vi "RT_VS50_Dynamics_DLR.vi"() -> ()   [LabVIEW 2017]
uses:
  <vilib>/Platform/TimedLoop/XDataNode/timing_clust.ctl
  <vilib>/Platform/TimedLoop/XDataNode/nitl_modes.ctl
  <vilib>/Platform/TimedLoop/XDataNode/wakeup.ctl
  <vilib>/Analysis/coordinate.llb/Euler Rotation Order.ctl
  <vilib>/Analysis/baseanly.llb/Real A x B.vi
  <vilib>/Utility/file.llb/Read Delimited Spreadsheet (DBL).vi
  <vilib>/Analysis/Matrix/Numeric/Conversions/Array To Matrix - RA.vi
  <vilib>/Analysis/Matrix/Numeric/Conversions/Array To Matrix - RA2.vi
  <vilib>/Analysis/Matrix/Numeric/Conversions/Matrix To Array - RM.vi
  <vilib>/platform/TimedLoop/XDataNode/XDataNode.xnode
  <vilib>/Platform/TimedLoop/XDataNode/XDNodeRunTimeDep.lvlib
  <vilib>/Analysis/Matrix/NI_Matrix.lvlib
  <vilib>/Analysis/NI_AALBase.lvlib
  <vilib>/Analysis/NI_AALPro.lvlib
panel:
  out "M_beta":dbl
  out "M_alpha":dbl
  out "TVA_cmd [rad]":dbl[](array[numeric])
  in  "TVA_y [º]":dbl=-0.01 format="%#_13g"
  in  "TVA_p [º]":dbl=-0.01 format="%#_13g"
  out "Sref [m^2]":dbl
  out "MAd [Nm]":dbl[](array[numeric])
  out "MA_f [Nm]":dbl[](array[numeric])
  out "TVA_b":dbl[](array[numeric])
  out "P(i) [m/s]":dbl[](array[numeric])
  out "MFE_b":dbl[](array[numeric])
  out "Euler Angles [º]":cluster{"phi":dbl, "theta":dbl, "psi":dbl}
  out "Euler Angles [rad]":cluster{"phi":dbl, "theta":dbl, "psi":dbl}
  out "Waveform Chart":T1(graph)
  out "alt(i)":dbl
  out "alt(i+1)":dbl
  out "lon(i)":dbl
  out "latd(i)":dbl
  out "lon(i+1)":dbl
  out "latd(i+1)":dbl
  out "R_lh [m]":dbl
  out "R_l [m]":dbl
  out "L_C [rad]":dbl
  out "D_l [rad]":dbl
  out "W_b(i) [º/s]":dbl[](array[numeric])
  out "q(i)":dbl[](array[numeric])
  out "W(i)":dbl[](array[numeric])
  out "V(i+1)":dbl[](array[numeric])
  out "V(i) [m/s]":dbl[](array[numeric])
  out "W(i+1)":dbl[](array[numeric])
  out "q(i+1)":dbl[](array[numeric])
  out "z(i)":dbl[](array[numeric])
  out "y(i)":dbl[](array[numeric])
  out "x(i)":dbl[](array[numeric])
  out "z(i+1)":dbl[](array[numeric])
  out "y(i+1)":dbl[](array[numeric])
  out "x(i+1)":dbl[](array[numeric])
  out "t [s]":dbl
  out "dt[s]":dbl
  in  "Tempo total de simulação":i32=85
  out "ang_acc [rad/s^2]":dbl[](array[numeric])
  out "acc [m/s^2]":dbl[](array[numeric])
  out "MFA [Nm]":dbl[](array[numeric])
  out "MFE [Nm]":dbl[](array[numeric])
  out "Mco [Nm]":dbl[](array[numeric])
  out "Fco [N]":dbl[](array[numeric])
  out "FA [N]":dbl[](array[numeric])
  out "FG_b [N]":dbl[](array[numeric])
  out "FG [N]":dbl[](array[numeric])
  out "FE [N]":dbl[](array[numeric])
  out "FE_b [N]":dbl[](array[numeric])
  out "AoA_yaw [rad]":dbl
  out "AoA_pitch [rad]":dbl
  out "Iteration Duration":i64(graph)
  out "Patm [Pa]":dbl
  out "Pdin [Pa]":dbl
  out "Nzl_S [m^2]":dbl
  out "Data":dbl[][](array[numeric])
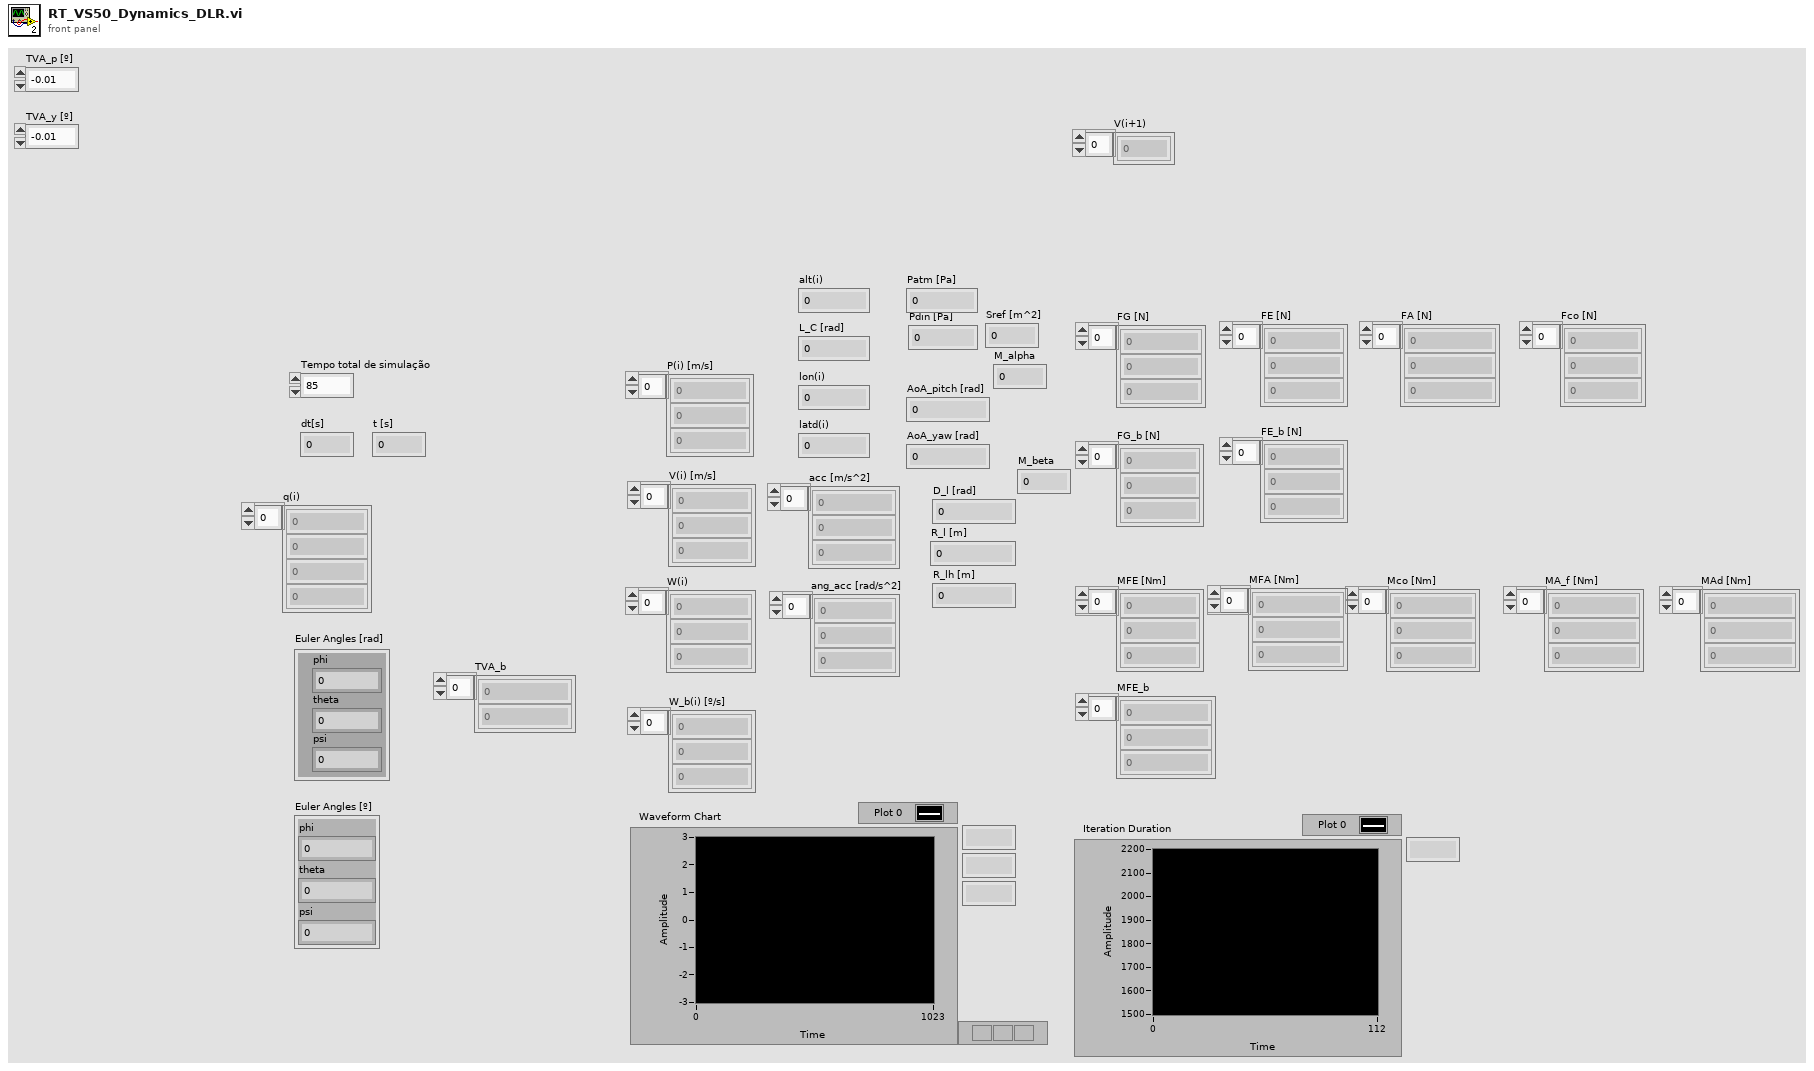
[diagram p1: front panel]
types:
  T1 = cluster{"Real Matrix Element":dbl, "Real Matrix Element":dbl, "Real Matrix Element":dbl}
  T2 = typedef "XDNodeRunTimeDep.lvlib/timing_clust.ctl" = cluster{"Expected End [f-1]":u64, "Actual End [f-1]":u64, "Finished Late? [f-1]":bool, "Expected End [i-1]":u64, "Actual End [i-1]":u64, "Finished Late? [i-1]":bool, "Expected Start [i]":u64, "Actual Start [i]":u64, "Expected Start [f]":u64, "Actual Start [f]":u64, "Source Name":string, "Structure Name":string, "Period":i64, "Deadline":i64, "Offset":i64, "Start":i64, "Priority":i32, "Timeout":i32, "Mode":T3, "Wakeup Reason":T4, "Error":errorcluster, "Source Type":string, "Secondary Source Type":string, "Global End Time":u64, "Global Start Time":u64, "Frame Duration":u64, "Iteration Duration":u64, "Assigned CPU":i32, "I/O Scan Engine Mode":u32}
  T3 = typedef "XDNodeRunTimeDep.lvlib/nitl_modes.ctl" = enum32{"No Change", "Process missed periods, maintain original phase", "Discard missed periods, maintain original phase", "Process missed periods, ignore original phase", "Discard missed periods, ignore original phase"}
  T4 = typedef "XDNodeRunTimeDep.lvlib/wakeup.ctl" = enum32{"Normal", "Aborted", "Asynchronous wakeup", "Timing source error", "Timed loop error", "Timeout"}
  T5 = typedef "NI_AALPro.lvlib/Euler Rotation Order.ctl" = u16
  T6 = typedef "NI_Matrix.lvlib/RealMatrix.ctl" = dbl[][]
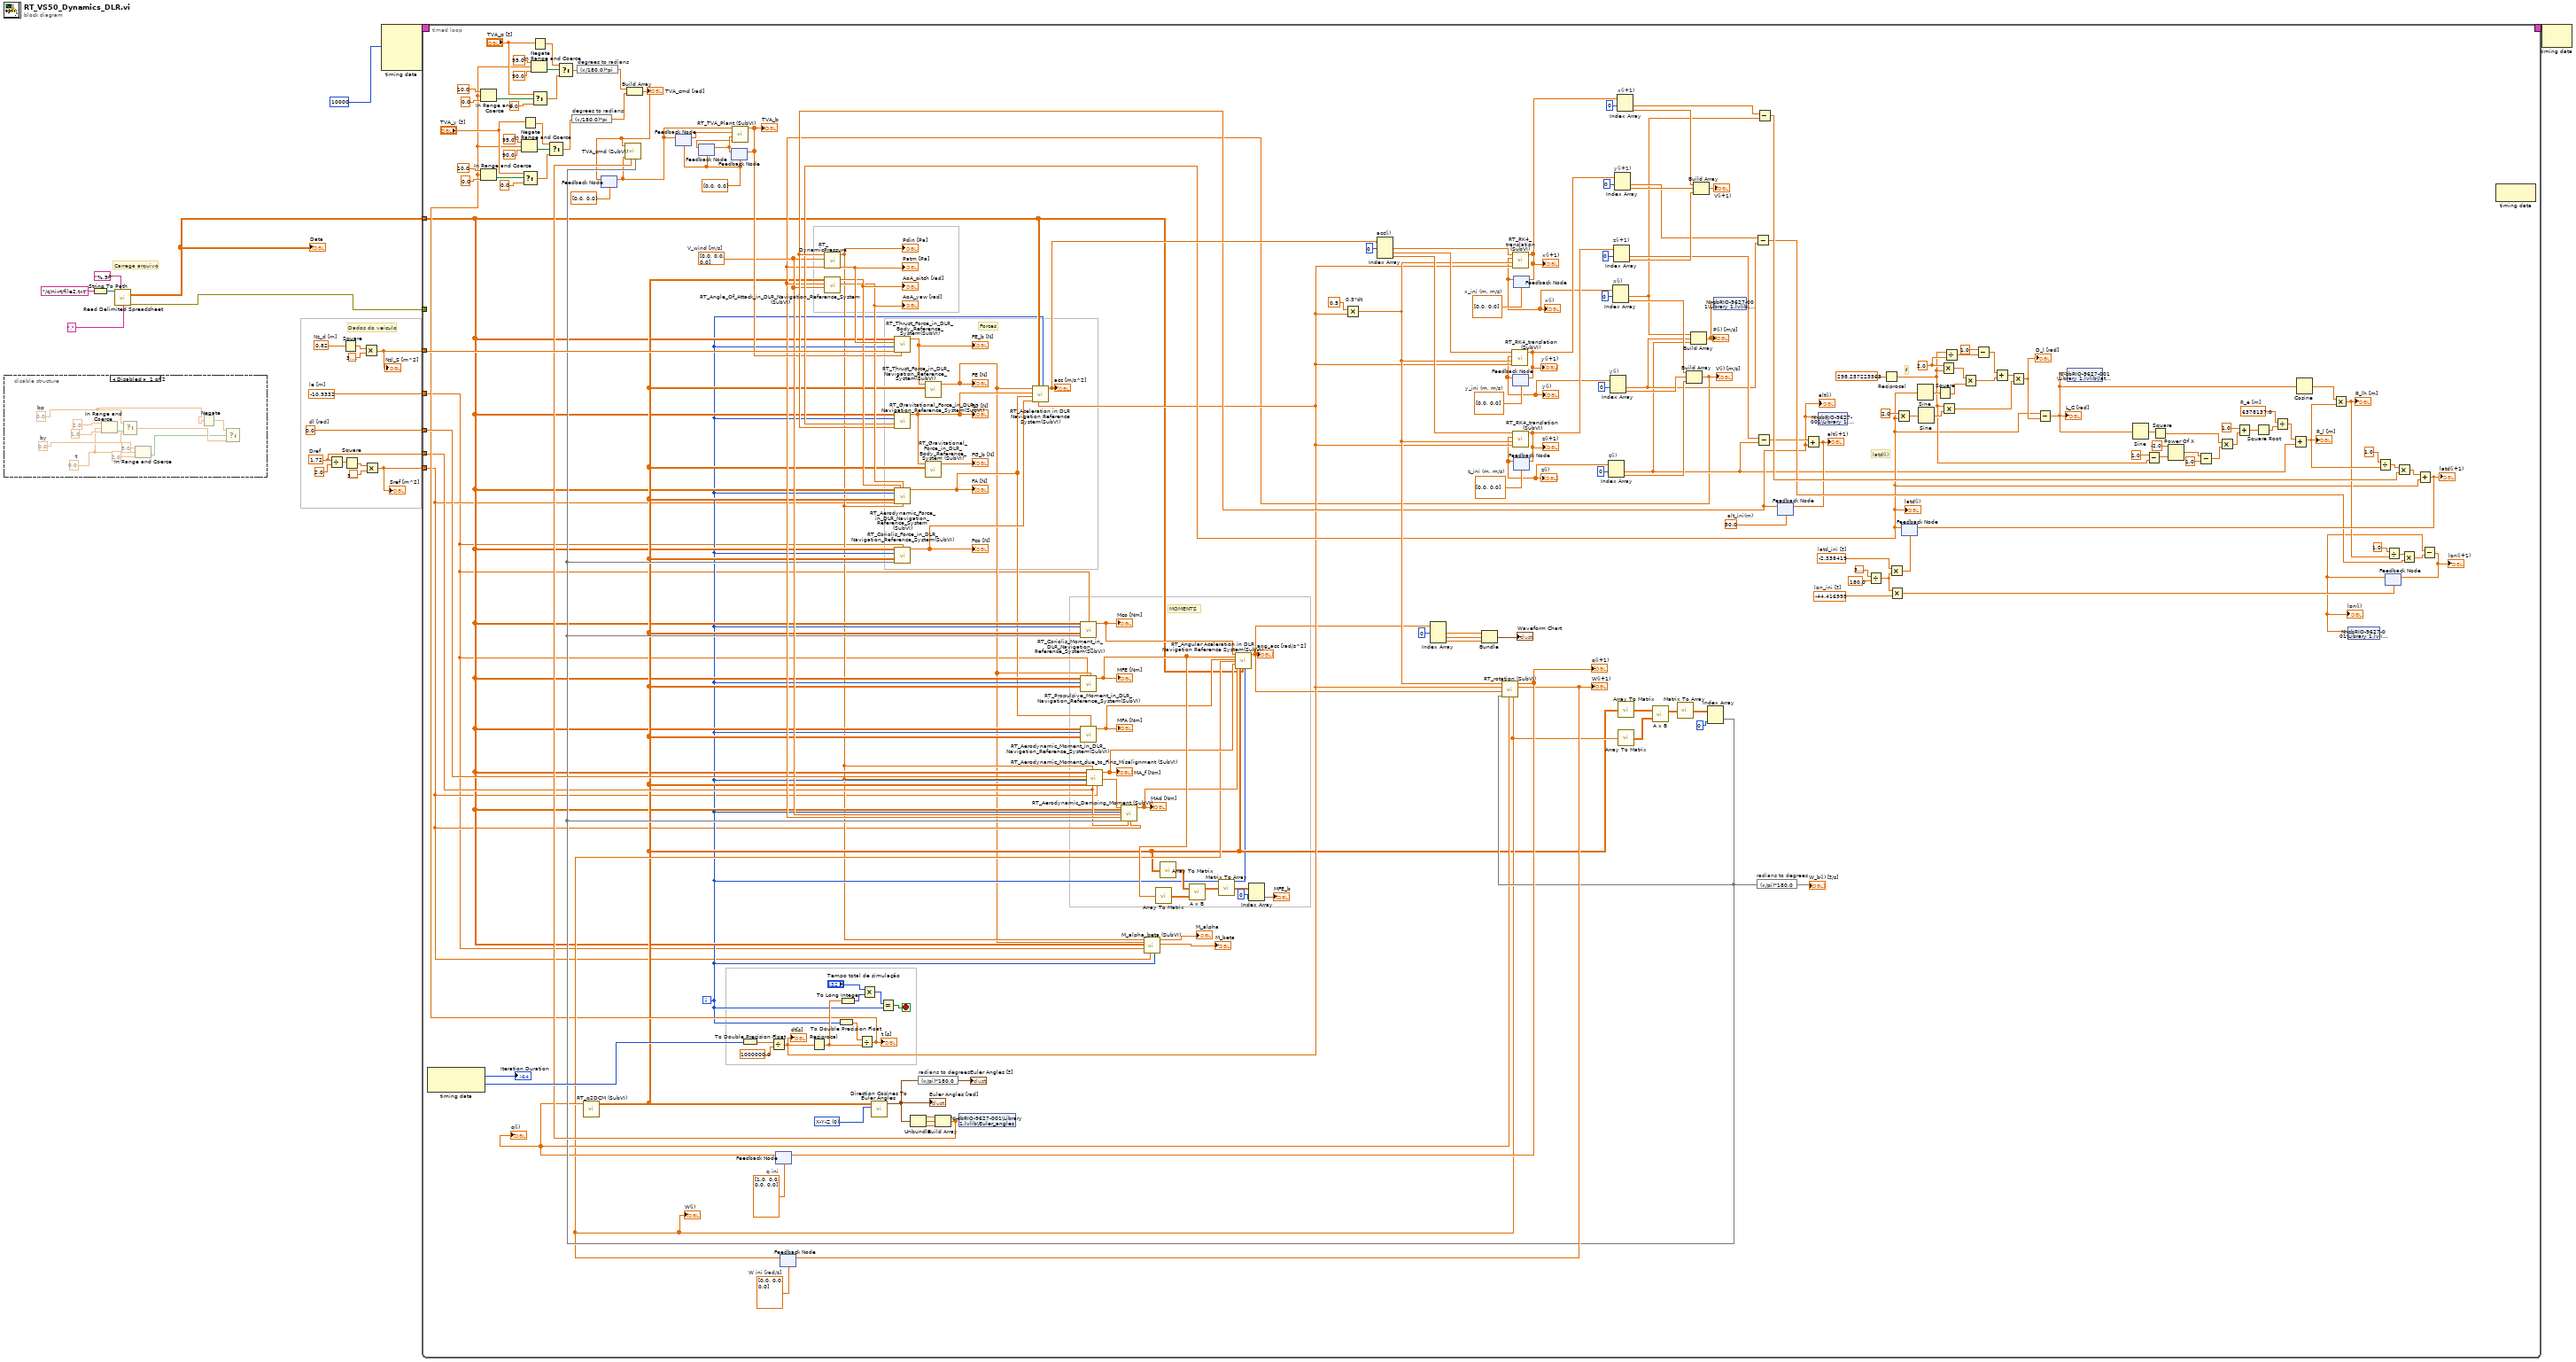
[diagram p0: block diagram]
diagram:
  w1 = 1.72  # Dref
  w7 = 0.0  # dl [rad]
  w14 = 0.82  # Nz_d [m]
  w15 = -10.9332  # le [m]
  # "Carrega arquivo"
  # "Dados do veículo"
  n1 = disable-structure shown="Disabled" {
    frame Disabled {
      w23 = 0.0  # t
      w24 = 0.0  # by
      w22 = 0.0  # bp
      n2 = In Range and Coerce(upper limit=2.0, x=w23, lower limit=1.0 ("y")) -> (In Range?=w31:bool)  [unwired: 1 out]
      n3 = Select(t=w22, s=w31, f=w24) -> (s? t:f=w27:dbl)
      n4 = In Range and Coerce(upper limit=3.0, x=w23, lower limit=2.0) -> (In Range?=w25:bool)  [unwired: 1 out]
      n5 = Negate(x=w22) -> (-x=w28:dbl)
      n6 = Select(t=w28, s=w25, f=w27) -> ()  [unwired: 1 out]
    }
    frame Enabled {
    }
  }
  n7 = String To Path(string="/c/ni-rt/file2.txt") -> (path=w18:path)
  n8 = call-poly <vilib>:"Read Delimited Spreadsheet.vi"("file path (dialog if empty)"=w18, "format (%.3f)"="%.9f", "delimiter (\\t)"="," ("delimiter (\\t)")) -> ("all rows"=w8:dbl[][], "error out"=w11:errorcluster)  [unwired: 7 in, 4 out]
  "Data" <- w8
  n9 = Divide(x=w1, y=2.0) -> (x/y=w3:dbl)
  n10 = Square(x=w14) -> (x^2=w17:dbl)
  n11 = Square(x=w3) -> (x^2=w4:dbl)
  n12 = Multiply(x=w17, y=3.141592653589793) -> (x*y=w13:dbl)
  "Nzl_S [m^2]" <- w13
  n13 = Multiply(x=w4, y=3.141592653589793) -> (x*y=w2:dbl)
  "Sref [m^2]" <- w2
  n14 = node-c288(i64 10000 ("Period")) -> (w21:T2)  [unwired: 3 in]
  n15 = timed-loop {
    timing: w21 -> [_]
    timing-out: [_] -> w20
    tunnel: w8 -> [w41]
    tunnel: w15 -> [w35]
    tunnel: w13 -> [w225]
    tunnel: w11 -> [_]
    tunnel: w7 -> [w83]
    tunnel: w2 -> [w38]
    tunnel: w1 -> [w43]
    i -> [w40]
    stop <- w227 stop-if-true
    w115 = T5 0 items=["X-Y-Z", "X-Z-Y", "Y-X-Z", "Y-Z-X", "Z-X-Y", "Z-Y-X", "X-Y-X", "X-Z-X", "Y-X-Y", "Y-Z-Y", "Z-X-Z", "Z-Y-Z"] ("rotation order")
    w89 = dbl[] [0.0, 0.0] ("TVA_b")
    w130 = 50.0  # alt_ini(m)
    w170 = 2.0 ("x")
    w150 = 6378137.0  # R_e [m]
    w82 = dbl[] [0.0, 0.0, 0.0]  # V_wind [m/s]
    w181 = -44.416995  # lon_ini [º]
    w183 = -2.338419  # latd_ini [º]
    w206 = dbl[] [0.0, 0.0]  # z_ini (m, m/s)
    w126 = dbl[] [0.0, 0.0, 0.0]  # W ini [rad/s]
    w207 = dbl[] [0.0, 0.0]  # y_ini (m, m/s)
    w210 = dbl[] [0.0, 0.0]  # x_ini (m, m/s)
    w127 = dbl[] [1.0, 0.0, 0.0, 0.0]  # q ini
    # "MOMENTS"
    # "Forces"
    # "f"
    # "latd(i)"
    n16 = node-c288() -> (→"Iteration Duration":i64, w216:i64)  [unwired: 1 in]
    n17 = Negate(x="TVA_y [º]") -> (-x=w49:dbl)
    n18 = Negate(x="TVA_p [º]") -> (-x=w70:dbl)
    n19 = feedback #1(dbl[] [0.0, 0.0] ("TVA_cmd")) -> (w44:dbl[])
    n20 = feedback #2(w89) -> (w88:dbl[])
    n21 = feedback-in #2(w44) -> ()
    n22 = feedback #3(w89) -> (w85:dbl[])
    n23 = feedback #4(w89) -> (w86:dbl[])
    n24 = feedback-in #3(w86) -> ()
    n25 = call "RT_TVA_Plant (SubVI).vi"("TVA_b(i-2)"=w85, "TVA_b(i-1)"=w86, "TVA_cmd (i-2) [rad]"=w88, "TVA_cmd (i-1) [rad]"=w44) -> ("TVA_b"=w87:dbl[])  [unwired: 7 in]
    "TVA_b" <- w87
    n26 = feedback-in #4(w87) -> ()
    n27 = To Double Precision Float(number=w216) -> (double precision float=w215:dbl)
    n28 = Divide(x=w215, y=1000000.0) -> (x/y=w117:dbl)
    "dt[s]" <- w117
    n29 = feedback #5(w127) -> (w79:dbl[])
    "q(i)" <- w79
    n30 = call "RT_q2DCM (SubVI).vi"("Quaternion"=w79) -> ("DCM"=w42:dbl[][])  [unwired: 10 in]
    n31 = feedback #6(w126) -> (w72:dbl[])
    "W(i)" <- w72
    n32 = Reciprocal(x=w117) -> (1/x=w187:dbl)
    n33 = To Double Precision Float(number=w40) -> (double precision float=w186:dbl)
    n34 = To Long Integer(number=w187) -> (32bit integer=w213:i32)
    n35 = Divide(x=w186, y=w187) -> (x/y=w46:dbl)
    "t [s]" <- w46
    n36 = In Range and Coerce(upper limit=10.0, x=w46, lower limit=0.0) -> (In Range?=w64:bool)  [unwired: 1 out]
    n37 = In Range and Coerce(upper limit=10.0, x=w46, lower limit=0.0) -> (In Range?=w52:bool)  [unwired: 1 out]
    n38 = In Range and Coerce(upper limit=95.0, x=w46, lower limit=90.0) -> (In Range?=w51:bool)  [unwired: 1 out]
    n39 = Select(t="TVA_y [º]", s=w52, f=0.0 ("t")) -> (s? t:f=w50:dbl)
    n40 = In Range and Coerce(upper limit=95.0, x=w46, lower limit=90.0) -> (In Range?=w65:bool)  [unwired: 1 out]
    n41 = Select(t="TVA_p [º]", s=w64, f=0.0 ("t")) -> (s? t:f=w67:dbl)
    n42 = Select(t=w49, s=w51, f=w50) -> (s? t:f=w47:dbl)
    n43 = Select(t=w70, s=w65, f=w67) -> (s? t:f=w66:dbl)
    n44 = expression code="(x/180.0)*pi" "degrees to radians"(w47) -> (w69:dbl)
    n45 = expression code="(x/180.0)*pi" "degrees to radians"(w66) -> (w68:dbl)
    n46 = Build Array(w68, w69) -> (w45:dbl[])
    "TVA_cmd [rad]" <- w45
    n47 = feedback-in #1(w45) -> ()
    n48 = Multiply(x="Tempo total de simulação", y=w213) -> (x*y=w228:i32)
    n49 = call <vilib>:"Direction Cosines To Euler Angles.vi"("rotation order"=w115, "Direction Cosines"=w42) -> ("Euler Angles"=w111:cluster{"phi":dbl, "theta":dbl, "psi":dbl})  [unwired: 8 in, 1 out]
    "Euler Angles [rad]" <- w111
    n50 = Equal?(x=w228, y=w40) -> (x = y?=w227:bool)
    n51 = Unbundle(w111) -> ("phi"=w114:dbl, "theta"=w112:dbl, "psi"=w113:dbl)
    n52 = expression code="(x/pi)*180.0" "radians to degrees"(w111) -> (→"Euler Angles [º]":cluster{"phi":dbl, "theta":dbl, "psi":dbl})
    n53 = Build Array(w114, w112, w113) -> (w90:dbl[])
    n54 = shared-variable "NI-sbRIO-9627-001\\Library 1.lvlib\\Euler_angles"(w90) -> ()  [unwired: 1 in, 1 out]
    n55 = call-poly <vilib>:"Array To Matrix.vi"("Real 2D Array"=w42) -> ("Real Matrix"=w98:T6)
    n56 = Multiply "0.5*dt"(x=0.5, y=w117) -> (x*y=w204:dbl)
    n57 = feedback #7(w207) -> (w96:dbl[])
    "y(i)" <- w96
    n58 = feedback #8(w210) -> (w97:dbl[])
    "x(i)" <- w97
    n59 = feedback #9(w206) -> (w95:dbl[])
    "z(i)" <- w95
    n60 = Index Array "z(i)"(array=w95, index #1=0 ("index")) -> (element #1=w92:dbl, element #2=w116:dbl)  [unwired: 1 in]
    n61 = Index Array "y(i)"(array=w96, index #1=0 ("index")) -> (element #1=w93:dbl, element #2=w198:dbl)  [unwired: 1 in]
    n62 = Index Array "x(i)"(array=w97, index #1=0 ("index")) -> (element #1=w94:dbl, element #2=w199:dbl)  [unwired: 1 in]
    n63 = call-poly <vilib>:"Array To Matrix.vi"("Real 2D Array"=w42) -> ("Real Matrix"=w125:T6)
    n64 = call-poly <vilib>:"Array To Matrix.vi"("Real 1D Array"=w72) -> ("Real Matrix (Column Vector)"=w124:T6)
    n65 = call-poly <vilib>:"A x B.vi"("B"=w124, "A"=w125) -> ("A x B"=w122:T6)  [unwired: 1 out]
    n66 = call-poly <vilib>:"Matrix To Array.vi"("Real Matrix"=w122) -> ("Real 2D Array"=w123:dbl[][])
    n67 = Build Array(w199, w198, w116) -> (w81:dbl[])
    "V(i) [m/s]" <- w81
    n68 = call "RT_Angle_Of_Attack_in_DLR_Navigation_Reference_System (SubVI).vi"("V_wind (m/s)"=w82, "V (m/s)"=w81, "DCM"=w42) -> ("AoA_yaw (rad)"=w221:dbl, "AoA_pitch (rad)"=w222:dbl)  [unwired: 7 in]
    "AoA_pitch [rad]" <- w222
    "AoA_yaw [rad]" <- w221
    n69 = Build Array(w94, w93, w92) -> (w71:dbl[])
    "P(i) [m/s]" <- w71
    n70 = Index Array(array=w123, index (col)=0 ("index (row)")) -> (element=w80:dbl[])  [unwired: 1 in]
    n71 = call "TVA_cmd (SubVI).vi"("W_b [rad/s]"=w80, "Angles [rad]"=w90, "TVA_old [rad]"=w44, "TVA_cmd [rad]"=w45) -> ()  [unwired: 6 in, 2 out]
    n72 = call "RT_Coriolis_Force_in_DLR_Navigation_Reference_System(SubVI).vi"("Data"=w41, "le (m) in"=w35, "i"=w40, "DCM"=w42, "W_b (rad/s)"=w80) -> ("Fco (N)"=w220:dbl[])  [unwired: 10 in]
    "Fco [N]" <- w220
    n73 = call "RT_Coriolis_Moment_in_DLR_Navigation_Reference_System(SubVI).vi"("Data"=w41, "le (m) in"=w35, "i"=w40, "DCM"=w42, "W_b (rad/s) in"=w80) -> ("Mco (Nm)"=w77:dbl[])  [unwired: 10 in]
    "Mco [Nm]" <- w77
    n74 = shared-variable "NI-sbRIO-9627-001\\Library 1.lvlib\\Pos"(w71) -> ()  [unwired: 1 in, 1 out]
    n75 = expression code="(x/pi)*180.0" "radians to degrees"(w80) -> (→"W_b(i) [º/s]":dbl[])
    n76 = feedback #10(w130) -> (w120:dbl)
    "alt(i)" <- w120
    n77 = call "RT_DynamicPressure.vi"("V (m/s)"=w81, "V_wind (m/s)"=w82, "h (m)"=w120) -> ("Patm (Pa)"=w223:dbl, "Pdin"=w39:dbl)  [unwired: 7 in]
    "Pdin [Pa]" <- w39
    "Patm [Pa]" <- w223
    n78 = call "RT_Thrust_Force_in_DLR_Body_Reference_System(SubVI).vi"("TVA_b(i)"=w87, "Nzl_S"=w225, "i"=w40, "Patm (Pa)"=w223, "Data"=w41) -> ("FE_b"=w104:dbl[])  [unwired: 6 in]
    "FE_b [N]" <- w104
    n79 = call "RT_Aerodynamic_Force_in_DLR_Navigation_Reference_System (SubVI).vi"("Data"=w41, "AoA_pitch (rad)"=w222, "AoA_yaw (rad)"=w221, "i"=w40, "DCM"=w42, "Sref [m^2]"=w38, "Pdin"=w39) -> ("FA"=w37:dbl[])  [unwired: 8 in]
    "FA [N]" <- w37
    n80 = call "RT_Thrust_Force_in_DLR_Navigation_Reference_System(SubVI).vi"("DCM"=w42, "FE_b"=w104) -> ("FE"=w36:dbl[])  [unwired: 8 in]
    "FE [N]" <- w36
    n81 = call "RT_Propulsive_Moment_in_DLR_Navigation_Reference_System(SubVI).vi"("FE"=w36, "le (m) in"=w35, "DCM"=w42, "i"=w40, "Data"=w41) -> ("MFE (Nm)"=w76:dbl[])  [unwired: 6 in]
    "MFE [Nm]" <- w76
    n82 = call "RT_Aerodynamic_Moment_in_DLR_Navigation_Reference_System(SubVI).vi"("FA"=w37, "DCM"=w42, "i"=w40, "Data"=w41) -> ("MFA (Nm)"=w75:dbl[])  [unwired: 7 in]
    "MFA [Nm]" <- w75
    n83 = call "RT_Aerodynamic_Moment_due_to_Fins_Misalignment (SubVI).vi"("Sref [m^2]"=w38, "Dref"=w43, "Pdin [Pa]"=w39, "DCM"=w42, "i"=w40, "dl [rad] in"=w83, "Data"=w41) -> ("MA_f"=w74:dbl[])  [unwired: 4 in]
    "MA_f [Nm]" <- w74
    n84 = call "RT_Aerodynamic_Damping_Moment (SubVI).vi"("Pdin [Pa]"=w39, "Data"=w41, "i"=w40, "V_wind [m/s]"=w82, "V(i) [m/s]"=w81, "W_b(i) [º/s]"=w80, "Dref"=w43, "Sref [m^2]"=w38) -> ("MAd"=w73:dbl[])  [unwired: 11 in]
    "MAd [Nm]" <- w73
    n85 = call "M_alpha_beta (SubVI).vi"("i"=w40, "Sref"=w38, "FE [N]"=w36, "le [m]"=w35, "Data"=w41, "Pdin [Pa]"=w39) -> ("M_beta"=→"M_beta":dbl, "M_alpha"=→"M_alpha":dbl)  [unwired: 4 in]
    n86 = call-poly <vilib>:"Array To Matrix.vi"("Real 1D Array"=w76) -> ("Real Matrix (Column Vector)"=w103:T6)
    n87 = call-poly <vilib>:"A x B.vi"("B"=w103, "A"=w98) -> ("A x B"=w101:T6)  [unwired: 1 out]
    n88 = call-poly <vilib>:"Matrix To Array.vi"("Real Matrix"=w101) -> ("Real 2D Array"=w102:dbl[][])
    n89 = call "RT_Angular Aceleration in DLR Navigation Reference System(SubVI).vi"("Mco (Nm)"=w77, "MFE (Nm)"=w76, "MFA (Nm)"=w75, "W (rad/s)"=w72, "MA_f [Nm]"=w74, "MAd [Nm]"=w73, "DCM"=w42, "Data"=w41, "i"=w40) -> ("ang_acc"=w78:dbl[])  [unwired: 10 in]
    "ang_acc [rad/s^2]" <- w78
    n90 = Index Array(array=w102, index (col)=0 ("index (row)")) -> (element=→"MFE_b":dbl[])  [unwired: 1 in]
    n91 = Index Array(array=w78, index #1=0 ("index")) -> (element #1=w108:dbl, element #2=w106:dbl, element #3=w107:dbl)  [unwired: 2 in]
    n92 = Bundle("Real Matrix Element"=w108, "Real Matrix Element"=w106, "Real Matrix Element"=w107) -> (→"Waveform Chart":T1)  [unwired: 1 in]
    n93 = call "RT_rotation (SubVI).vi"("W(i) (rad/s) in"=w72, "q(i) in"=w79, "W_b(i)"=w80, "ang_acc"=w78, "dt"=w117, "dt*0.5"=w204) -> ("W(i+1)"=w84:dbl[], "q(i+1)"=w203:dbl[])  [unwired: 4 in]
    "q(i+1)" <- w203
    "W(i+1)" <- w84
    n94 = feedback-in #5(w203) -> ()
    n95 = feedback-in #6(w84) -> ()
    n96 = shared-variable "NI-sbRIO-9627-001\\Library 1.lvlib\\alt"(w120) -> ()  [unwired: 1 in, 1 out]
    n97 = Divide(x=3.141592653589793, y=180.0) -> (x/y=w182:dbl)
    n98 = Reciprocal(x=298.257223563) -> (1/x=w161:dbl)
    n99 = Multiply(x=w183, y=w182) -> (x*y=w179:dbl)
    n100 = Multiply(x=w182, y=w181) -> (x*y=w178:dbl)
    n101 = feedback #11(w179) -> (w119:dbl)
    "latd(i)" <- w119
    n102 = call "RT_Gravitational_Force_in_DLR_Navigation_Reference_System(SubVI).vi"("Data"=w41, "i"=w40, "latd (rad)"=w119, "alt (m)"=w120) -> ("FG_d"=w218:dbl[])  [unwired: 10 in, 1 out]
    "FG [N]" <- w218
    n103 = call "RT_Gravitational_Force_in_DLR_Body_Reference_System (SubVI).vi"("DCM"=w42, "FG_d"=w218) -> ("FG_b"=→"FG_b [N]":dbl[])  [unwired: 9 in]
    n104 = call "RT_Aceleration in DLR Navigation Reference System(SubVI).vi"("i"=w40, "dt(s)"=w117, "Data"=w41, "Fco (N)"=w220, "FA"=w37, "FG"=w218, "FE"=w36) -> ("acc"=w212:dbl[])  [unwired: 4 in]
    "acc [m/s^2]" <- w212
    n105 = Index Array "acc(i)"(array=w212, index #1=0 ("index")) -> (element #1=w209:dbl, element #2=w208:dbl, element #3=w205:dbl)  [unwired: 2 in]
    n106 = call "RT_RK4_translation (SubVI).vi"("dt"=w117, "dt*0.5"=w204, "x(i)"=w96, "accx"=w208) -> ("x(i+1)"=w193:dbl[])  [unwired: 7 in]
    "y(i+1)" <- w193
    n107 = call "RT_RK4_translation (SubVI).vi"("dt"=w117, "dt*0.5"=w204, "x(i)"=w97, "accx"=w209) -> ("x(i+1)"=w192:dbl[])  [unwired: 7 in]
    "x(i+1)" <- w192
    n108 = feedback-in #7(w193) -> ()
    n109 = call "RT_RK4_translation (SubVI).vi"("dt"=w117, "dt*0.5"=w204, "x(i)"=w95, "accx"=w205) -> ("x(i+1)"=w194:dbl[])  [unwired: 7 in]
    "z(i+1)" <- w194
    n110 = feedback-in #8(w192) -> ()
    n111 = feedback-in #9(w194) -> ()
    n112 = Index Array "z(i+1)"(array=w194, index #1=0 ("index")) -> (element #1=w133:dbl, element #2=w188:dbl)  [unwired: 1 in]
    n113 = Index Array "y(i+1)"(array=w193, index #1=0 ("index")) -> (element #1=w138:dbl, element #2=w189:dbl)  [unwired: 1 in]
    n114 = Index Array "x(i+1)"(array=w192, index #1=0 ("index")) -> (element #1=w144:dbl, element #2=w190:dbl)  [unwired: 1 in]
    n115 = Build Array(w190, w189, w188) -> (→"V(i+1)":dbl[])
    n116 = Subtract(x=w138, y=w93) -> (x-y=w136:dbl)
    n117 = Subtract(x=w133, y=w92) -> (x-y=w132:dbl)
    n118 = Subtract(x=w144, y=w94) -> (x-y=w143:dbl)
    n119 = Add(x=w132, y=w120) -> (x+y=w131:dbl)
    "alt(i+1)" <- w131
    n120 = feedback-in #10(w131) -> ()
    n121 = Multiply(x=2.0, y=w119) -> (x*y=w176:dbl)
    n122 = Sine(x=w119) -> (sin(x)=w174:dbl)
    n123 = Sine(x=w176) -> (sin(x)=w175:dbl)
    n124 = Square(x=w174) -> (x^2=w172:dbl)
    n125 = Multiply(x=w170, y=w161) -> (x*y=w173:dbl)
    n126 = Multiply(x=w161, y=w175) -> (x*y=w165:dbl)
    n127 = Divide(x=w161, y=w170) -> (x/y=w169:dbl)
    n128 = Multiply(x=w173, y=w172) -> (x*y=w171:dbl)
    n129 = Subtract(x=1.0, y=w169) -> (x-y=w167:dbl)
    n130 = Add(x=w167, y=w171) -> (x+y=w166:dbl)
    n131 = Multiply(x=w166, y=w165) -> (x*y=w164:dbl)
    "D_l [rad]" <- w164
    n132 = Subtract(x=w119, y=w164) -> (x-y=w129:dbl)
    "L_C [rad]" <- w129
    n133 = shared-variable "NI-sbRIO-9627-001\\Library 1.lvlib\\lat_c"(w129) -> ()  [unwired: 1 in, 1 out]
    n134 = Sine(x=w129) -> (sin(x)=w163:dbl)
    n135 = Subtract(x=1.0, y=w161) -> (x-y=w159:dbl)
    n136 = Square(x=w163) -> (x^2=w156:dbl)
    n137 = Power Of X(1:w159, 2:-2.0 ("y")) -> (0:w157:dbl)
    n138 = Subtract(x=w157, y=1.0 ("x")) -> (x-y=w155:dbl)
    n139 = Multiply(x=w156, y=w155) -> (x*y=w154:dbl)
    n140 = Add(x=1.0, y=w154) -> (x+y=w152:dbl)
    n141 = Square Root(x=w152) -> (sqrt(x)=w151:dbl)
    n142 = Divide(x=w150, y=w151) -> (x/y=w149:dbl)
    n143 = Add(x=w149, y=w92) -> (x+y=w146:dbl)
    "R_l [m]" <- w146
    n144 = Cosine(x=w129) -> (cos(x)=w148:dbl)
    n145 = Multiply(x=w148, y=w146) -> (x*y=w139:dbl)
    "R_lh [m]" <- w139
    n146 = Divide(x=1.0, y=w146) -> (x/y=w145:dbl)
    n147 = feedback #12(w178) -> (w128:dbl)
    "lon(i)" <- w128
    n148 = shared-variable "NI-sbRIO-9627-001\\Library 1.lvlib\\lon"(w128) -> ()  [unwired: 1 in, 1 out]
    n149 = Divide(x=1.0, y=w139) -> (x/y=w137:dbl)
    n150 = Multiply(x=w145, y=w143) -> (x*y=w142:dbl)
    n151 = Multiply(x=w137, y=w136) -> (x*y=w135:dbl)
    n152 = Add(x=w142, y=w119) -> (x+y=w141:dbl)
    "latd(i+1)" <- w141
    n153 = feedback-in #11(w141) -> ()
    n154 = Subtract(x=w128, y=w135) -> (x-y=w134:dbl)
    "lon(i+1)" <- w134
    n155 = feedback-in #12(w134) -> ()
    n156 = node-c288() -> ()  [unwired: 1 in, 1 out]
  }
  n157 = node-c288(w20) -> ()  [unwired: 1 out]
